vi "EminemNumbToState.vi"(11 "StateNumber":dbl) -> (3 "M&M_State":T1=enum."13-AmpDone")   [LabVIEW 2023]
uses:
  EminemStatesEnum.ctl
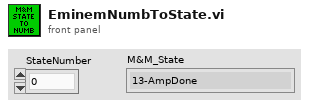
[diagram p1: front panel]
types:
  T1 = typedef "EminemStatesEnum.ctl" = enum16{"0-Init", "1-WaitForCmd", "2-Cancel", "3-ShootStart", "4-ShootRev", "5-RevUpStart", "6-ShootStartFeed&Timer", "7-ShootTimerOrSensorDone", "8-ShootDone", "9-AmpStart", "10-AmpUpToSpd?", "11-AmpStartFeed&Timer", "12-AmpTimerOrSensorDone", "13-AmpDone", "14-RevUpGetCmd"}
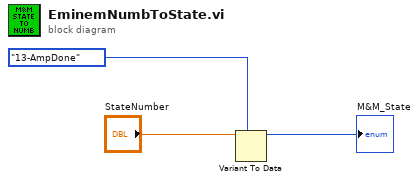
[diagram p0: block diagram]
diagram:
  n1 = Variant To Data(type=EminemStatesEnum."13-AmpDone" ("M&M_State 2"), Variant="StateNumber") -> (data=→"M&M_State":T1)  [unwired: 1 in, 1 out]
